vi "S2C_Access_Delete.vi"(8 "Error In":errorcluster, 10 "Condition":string, 11 "Table":string) -> (0 "Error Out":errorcluster)   [LabVIEW 2015]
uses:
  S2C_Access_Globals.vi
  <vilib>/addons/database/NI_Database_API.lvlib
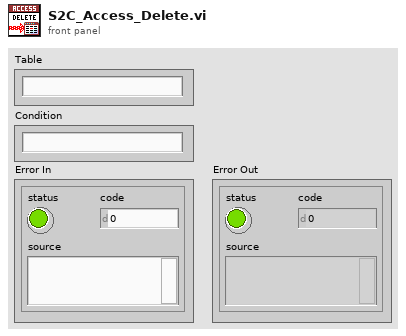
[diagram p1: front panel]
types:
  T1 = typedef "NI_Database_API.lvlib/Conn ObjectReference.ctl" = refnum<k1>
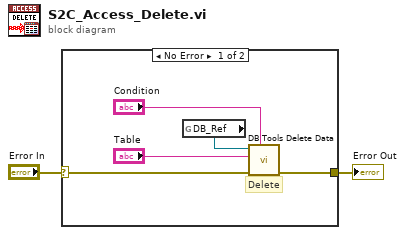
[diagram p0: block diagram]
diagram:
  n1 = case shown="No Error" "Error In" {
    selector: "Error In" -> [w7 w8]
    tunnel: [w6 w8] -> w1
    frame No Error {
      # "Delete"
      n2 = global read "S2C_Access_Globals.vi" "DB_Ref"() -> (w5:T1)
      n3 = call <vilib>:"DB Tools Delete Data.vi"("condition"="Condition", "error in (no error)"=w7, "table"="Table", "connection reference"=w5) -> ("error out"=w6:errorcluster)  [unwired: 6 in, 1 out]
    }
    frame Error {
    }
  }
  "Error Out" <- w1
